vi "RegisterPatchGenerator.vi"(8 "error in":errorcluster, 9 "reg patch file":path=path "C:/Users/liyao/Desktop/New Text Document.Reg", 11 "exe path":path=path "C:/Users/liyao/Desktop/LabVIEW-Version-Selector/Build/LabVIEW Version Selector.exe") -> (0 "error out":errorcluster, 3 "delimited string":string="Windows Registry Editor Version 5.00\n\n[HKEY_CLASSES_ROOT\\Applications\\LabVIEW Version Selector.exe]\n\n[HKEY_CLASSES_ROOT\\Applications\\LabVIEW Version Selector.exe\\shell]\n\n[HKEY_CLASSES_ROOT\\Applications\\LabVIEW Version Selector.exe\\shell\\open]\n\n[HKEY_CLASSES_ROOT\\Applications\\LabVIEW Version Selector.exe\\shell\\open\\command]\n@=\"\\\"\"\"\" \"%1\"\"\\\" \\\"%1\\\"\"\n\n[HKEY_CURRENT_USER\\Software\\Classes\\Applications\\LabVIEW Version Selector.exe]\n\n[HKEY_CURRENT_USER\\Software\\Classes\\Applications\\LabVIEW Version Selector.exe\\shell]\n\n[HKEY_CURRENT_USER\\Software\\Classes\\Applications\\LabVIEW Version Selector.exe\\shell\\open]\n\n[HKEY_CURRENT_USER\\Software\\Classes\\Applications\\LabVIEW Version Selector.exe\\shell\\open\\command]\n@=\"\\\"\"\"\" \"%1\"\"\\\" \\\"%1\\\"\"\n\n[HKEY_CURRENT_USER\\Software\\Microsoft\\Windows\\CurrentVersion\\Explorer\\FileExts\\.lvproj\\OpenWithList]\n\"a\"=\"LabVIEW.exe\"\n\"b\"=\"LabVIEW Version Selector.exe\"\n\"MRUList\"=\"ba\"\n\n[HKEY_CURRENT_USER\\Software\\Microsoft\\Windows\\CurrentVersion\\Explorer\\FileExts\\.lvproj\\UserChoice]\n\"ProgId\"=\"Applications\\\\LabVIEW Version Selector.exe\"\n\n[HKEY_CLASSES_ROOT\\LabVIEWProject\r\n\\shell\\open\\command]\n@=\"\\\"\"\"\" \"%1\"\"\\\" \\\"%1\\\"\"\n\n[HKEY_LOCAL_MACHINE\\SOFTWARE\\Classes\\LabVIEWProject\r\n\\shell\\open\\command]\n@=hex(2):<HEXEXEPATH>\n\n[HKEY_CURRENT_USER\\Software\\Microsoft\\Windows\\CurrentVersion\\Explorer\\FileExts\\.lvlib\\OpenWithList]\n\"a\"=\"LabVIEW.exe\"\n\"b\"=\"LabVIEW Version Selector.exe\"\n\"MRUList\"=\"ba\"\n\n[HKEY_CURRENT_USER\\Software\\Microsoft\\Windows\\CurrentVersion\\Explorer\\FileExts\\.lvlib\\UserChoice]\n\"ProgId\"=\"Applications\\\\LabVIEW Version Selector.exe\"\n\n[HKEY_CLASSES_ROOT\\LabVIEWLabVIEW Library\r\n\\shell\\open\\command]\n@=\"\\\"\"\"\" \"%1\"\"\\\" \\\"%1\\\"\"\n\n[HKEY_LOCAL_MACHINE\\SOFTWARE\\Classes\\LabVIEWLabVIEW Library\r\n\\shell\\open\\command]\n@=hex(2):<HEXEXEPATH>\n\n[HKEY_CURRENT_USER\\Software\\Microsoft\\Windows\\CurrentVersion\\Explorer\\FileExts\\.lvlibp\\OpenWithList]\n\"a\"=\"LabVIEW.exe\"\n\"b\"=\"LabVIEW Version Selector.exe\"\n\"MRUList\"=\"ba\"\n\n[HKEY_CURRENT_USER\\Software\\Microsoft\\Windows\\CurrentVersion\\Explorer\\FileExts\\.lvlibp\\UserChoice]\n\"ProgId\"=\"Applications\\\\LabVIEW Version Selector.exe\"\n\n[HKEY_CLASSES_ROOT\\LabVIEWLabVIEW Packed Library\r\n\\shell\\open\\command]\n@=\"\\\"\"\"\" \"%1\"\"\\\" \\\"%1\\\"\"\n\n[HKEY_LOCAL_MACHINE\\SOFTWARE\\Classes\\LabVIEWLabVIEW Packed Library\r\n\\shell\\open\\command]\n@=hex(2):<HEXEXEPATH>\n\n[HKEY_CURRENT_USER\\Software\\Microsoft\\Windows\\CurrentVersion\\Explorer\\FileExts\\.vi\\OpenWithList]\n\"a\"=\"LabVIEW.exe\"\n\"b\"=\"LabVIEW Version Selector.exe\"\n\"MRUList\"=\"ba\"\n\n[HKEY_CURRENT_USER\\Software\\Microsoft\\Windows\\CurrentVersion\\Explorer\\FileExts\\.vi\\UserChoice]\n\"ProgId\"=\"Applications\\\\LabVIEW Version Selector.exe\"\n\n[HKEY_CLASSES_ROOT\\LabVIEWInstrument\r\n\\shell\\open\\command]\n@=\"\\\"\"\"\" \"%1\"\"\\\" \\\"%1\\\"\"\n\n[HKEY_LOCAL_MACHINE\\SOFTWARE\\Classes\\LabVIEWInstrument\r\n\\shell\\open\\command]\n@=hex(2):<HEXEXEPATH>\n\n[HKEY_CURRENT_USER\\Software\\Microsoft\\Windows\\CurrentVersion\\Explorer\\FileExts\\.llb\\OpenWithList]\n\"a\"=\"LabVIEW.exe\"\n\"b\"=\"LabVIEW Version Selector.exe\"\n\"MRUList\"=\"ba\"\n\n[HKEY_CURRENT_USER\\Software\\Microsoft\\Windows\\CurrentVersion\\Explorer\\FileExts\\.llb\\UserChoice]\n\"ProgId\"=\"Applications\\\\LabVIEW Version Selector.exe\"\n\n[HKEY_CLASSES_ROOT\\LabVIEWLibrary\r\n\\shell\\open\\command]\n@=\"\\\"\"\"\" \"%1\"\"\\\" \\\"%1\\\"\"\n\n[HKEY_LOCAL_MACHINE\\SOFTWARE\\Classes\\LabVIEWLibrary\r\n\\shell\\open\\command]\n@=hex(2):<HEXEXEPATH>\n\n[HKEY_CURRENT_USER\\Software\\Microsoft\\Windows\\CurrentVersion\\Explorer\\FileExts\\.ctl\\OpenWithList]\n\"a\"=\"LabVIEW.exe\"\n\"b\"=\"LabVIEW Version Selector.exe\"\n\"MRUList\"=\"ba\"\n\n[HKEY_CURRENT_USER\\Software\\Microsoft\\Windows\\CurrentVersion\\Explorer\\FileExts\\.ctl\\UserChoice]\n\"ProgId\"=\"Applications\\\\LabVIEW Version Selector.exe\"\n\n[HKEY_CLASSES_ROOT\\LabVIEWControl\r\n\\shell\\open\\command]\n@=\"\\\"\"\"\" \"%1\"\"\\\" \\\"%1\\\"\"\n\n[HKEY_LOCAL_MACHINE\\SOFTWARE\\Classes\\LabVIEWControl\r\n\\shell\\open\\command]\n@=hex(2):<HEXEXEPATH>\n\n[HKEY_CURRENT_USER\\Software\\Microsoft\\Windows\\CurrentVersion\\Explorer\\FileExts\\.lvclass\\OpenWithList]\n\"a\"=\"LabVIEW.exe\"\n\"b\"=\"LabVIEW Version Selector.exe\"\n\"MRUList\"=\"ba\"\n\n[HKEY_CURRENT_USER\\Software\\Microsoft\\Windows\\CurrentVersion\\Explorer\\FileExts\\.lvclass\\UserChoice]\n\"ProgId\"=\"Applications\\\\LabVIEW Version Selector.exe\"\n\n[HKEY_CLASSES_ROOT\\LabVIEWLabVIEW Class\r\n\\shell\\open\\command]\n@=\"\\\"\"\"\" \"%1\"\"\\\" \\\"%1\\\"\"\n\n[HKEY_LOCAL_MACHINE\\SOFTWARE\\Classes\\LabVIEWLabVIEW Class\r\n\\shell\\open\\command]\n@=hex(2):<HEXEXEPATH>\n\n[HKEY_CURRENT_USER\\Software\\Microsoft\\Windows\\CurrentVersion\\Explorer\\FileExts\\.vit\\OpenWithList]\n\"a\"=\"LabVIEW.exe\"\n\"b\"=\"LabVIEW Version Selector.exe\"\n\"MRUList\"=\"ba\"\n\n[HKEY_CURRENT_USER\\Software\\Microsoft\\Windows\\CurrentVersion\\Explorer\\FileExts\\.vit\\UserChoice]\n\"ProgId\"=\"Applications\\\\LabVIEW Version Selector.exe\"\n\n[HKEY_CLASSES_ROOT\\LabVIEWInstrumentTemplate\r\n\\shell\\open\\command]\n@=\"\\\"\"\"\" \"%1\"\"\\\" \\\"%1\\\"\"\n\n[HKEY_LOCAL_MACHINE\\SOFTWARE\\Classes\\LabVIEWInstrumentTemplate\r\n\\shell\\open\\command]\n@=hex(2):<HEXEXEPATH>\n\n[HKEY_CURRENT_USER\\Software\\Microsoft\\Windows\\CurrentVersion\\Explorer\\FileExts\\.xctl\\OpenWithList]\n\"a\"=\"LabVIEW.exe\"\n\"b\"=\"LabVIEW Version Selector.exe\"\n\"MRUList\"=\"ba\"\n\n[HKEY_CURRENT_USER\\Software\\Microsoft\\Windows\\CurrentVersion\\Explorer\\FileExts\\.xctl\\UserChoice]\n\"ProgId\"=\"Applications\\\\LabVIEW Version Selector.exe\"\n\n[HKEY_CLASSES_ROOT\\LabVIEWXControl\r\n\\shell\\open\\command]\n@=\"\\\"\"\"\" \"%1\"\"\\\" \\\"%1\\\"\"\n\n[HKEY_LOCAL_MACHINE\\SOFTWARE\\Classes\\LabVIEWXControl\r\n\\shell\\open\\command]\n@=hex(2):<HEXEXEPATH>\n\n[HKEY_CURRENT_USER\\Software\\Microsoft\\Windows\\CurrentVersion\\Explorer\\FileExts\\.lvtest\\OpenWithList]\n\"a\"=\"LabVIEW.exe\"\n\"b\"=\"LabVIEW Version Selector.exe\"\n\"MRUList\"=\"ba\"\n\n[HKEY_CURRENT_USER\\Software\\Microsoft\\Windows\\CurrentVersion\\Explorer\\FileExts\\.lvtest\\UserChoice]\n\"ProgId\"=\"Applications\\\\LabVIEW Version Selector.exe\"\n\n[HKEY_CLASSES_ROOT\\\\shell\\open\\command]\n@=\"\\\"\"\"\" \"%1\"\"\\\" \\\"%1\\\"\"\n\n[HKEY_LOCAL_MACHINE\\SOFTWARE\\Classes\\\\shell\\open\\command]\n@=hex(2):<HEXEXEPATH>\n\n[HKEY_CURRENT_USER\\Software\\Microsoft\\Windows\\CurrentVersion\\Explorer\\FileExts\\.lvvect\\OpenWithList]\n\"a\"=\"LabVIEW.exe\"\n\"b\"=\"LabVIEW Version Selector.exe\"\n\"MRUList\"=\"ba\"\n\n[HKEY_CURRENT_USER\\Software\\Microsoft\\Windows\\CurrentVersion\\Explorer\\FileExts\\.lvvect\\UserChoice]\n\"ProgId\"=\"Applications\\\\LabVIEW Version Selector.exe\"\n\n[HKEY_CLASSES_ROOT\\\\shell\\open\\command]\n@=\"\\\"\"\"\" \"%1\"\"\\\" \\\"%1\\\"\"\n\n[HKEY_LOCAL_MACHINE\\SOFTWARE\\Classes\\\\shell\\open\\command]\n@=hex(2):<HEXEXEPATH>\n\n[HKEY_CURRENT_USER\\Software\\Microsoft\\Windows\\CurrentVersion\\Explorer\\FileExts\\.lvsc\\OpenWithList]\n\"a\"=\"LabVIEW.exe\"\n\"b\"=\"LabVIEW Version Selector.exe\"\n\"MRUList\"=\"ba\"\n\n[HKEY_CURRENT_USER\\Software\\Microsoft\\Windows\\CurrentVersion\\Explorer\\FileExts\\.lvsc\\UserChoice]\n\"ProgId\"=\"Applications\\\\LabVIEW Version Selector.exe\"\n\n[HKEY_CLASSES_ROOT\\LabVIEW Statechart\r\n\\shell\\open\\command]\n@=\"\\\"\"\"\" \"%1\"\"\\\" \\\"%1\\\"\"\n\n[HKEY_LOCAL_MACHINE\\SOFTWARE\\Classes\\LabVIEW Statechart\r\n\\shell\\open\\command]\n@=hex(2):<HEXEXEPATH>\n\n[HKEY_CURRENT_USER\\Software\\Microsoft\\Windows\\CurrentVersion\\Explorer\\FileExts\\.LVCLASS\\OpenWithList]\n\"a\"=\"LabVIEW.exe\"\n\"b\"=\"LabVIEW Version Selector.exe\"\n\"MRUList\"=\"ba\"\n\n[HKEY_CURRENT_USER\\Software\\Microsoft\\Windows\\CurrentVersion\\Explorer\\FileExts\\.LVCLASS\\UserChoice]\n\"ProgId\"=\"Applications\\\\LabVIEW Version Selector.exe\"\n\n[HKEY_CLASSES_ROOT\\LabVIEWLabVIEW Class\r\n\\shell\\open\\command]\n@=\"\\\"\"\"\" \"%1\"\"\\\" \\\"%1\\\"\"\n\n[HKEY_LOCAL_MACHINE\\SOFTWARE\\Classes\\LabVIEWLabVIEW Class\r\n\\shell\\open\\command]\n@=hex(2):<HEXEXEPATH>\n\n[HKEY_CURRENT_USER\\Software\\Microsoft\\Windows\\CurrentVersion\\Explorer\\FileExts\\.lvr\\OpenWithList]\n\"a\"=\"LabVIEW.exe\"\n\"b\"=\"LabVIEW Version Selector.exe\"\n\"MRUList\"=\"ba\"\n\n[HKEY_CURRENT_USER\\Software\\Microsoft\\Windows\\CurrentVersion\\Explorer\\FileExts\\.lvr\\UserChoice]\n\"ProgId\"=\"Applications\\\\LabVIEW Version Selector.exe\"\n\n[HKEY_CLASSES_ROOT\\\\shell\\open\\command]\n@=\"\\\"\"\"\" \"%1\"\"\\\" \\\"%1\\\"\"\n\n[HKEY_LOCAL_MACHINE\\SOFTWARE\\Classes\\\\shell\\open\\command]\n@=hex(2):<HEXEXEPATH>\n\n[HKEY_CURRENT_USER\\Software\\Microsoft\\Windows\\CurrentVersion\\Explorer\\FileExts\\.lvrbt\\OpenWithList]\n\"a\"=\"LabVIEW.exe\"\n\"b\"=\"LabVIEW Version Selector.exe\"\n\"MRUList\"=\"ba\"\n\n[HKEY_CURRENT_USER\\Software\\Microsoft\\Windows\\CurrentVersion\\Explorer\\FileExts\\.lvrbt\\UserChoice]\n\"ProgId\"=\"Applications\\\\LabVIEW Version Selector.exe\"\n\n[HKEY_CLASSES_ROOT\\LabVIEWNXTRobotProject\r\n\\shell\\open\\command]\n@=\"\\\"\"\"\" \"%1\"\"\\\" \\\"%1\\\"\"\n\n[HKEY_LOCAL_MACHINE\\SOFTWARE\\Classes\\LabVIEWNXTRobotProject\r\n\\shell\\open\\command]\n@=hex(2):<HEXEXEPATH>")   [LabVIEW 2014]
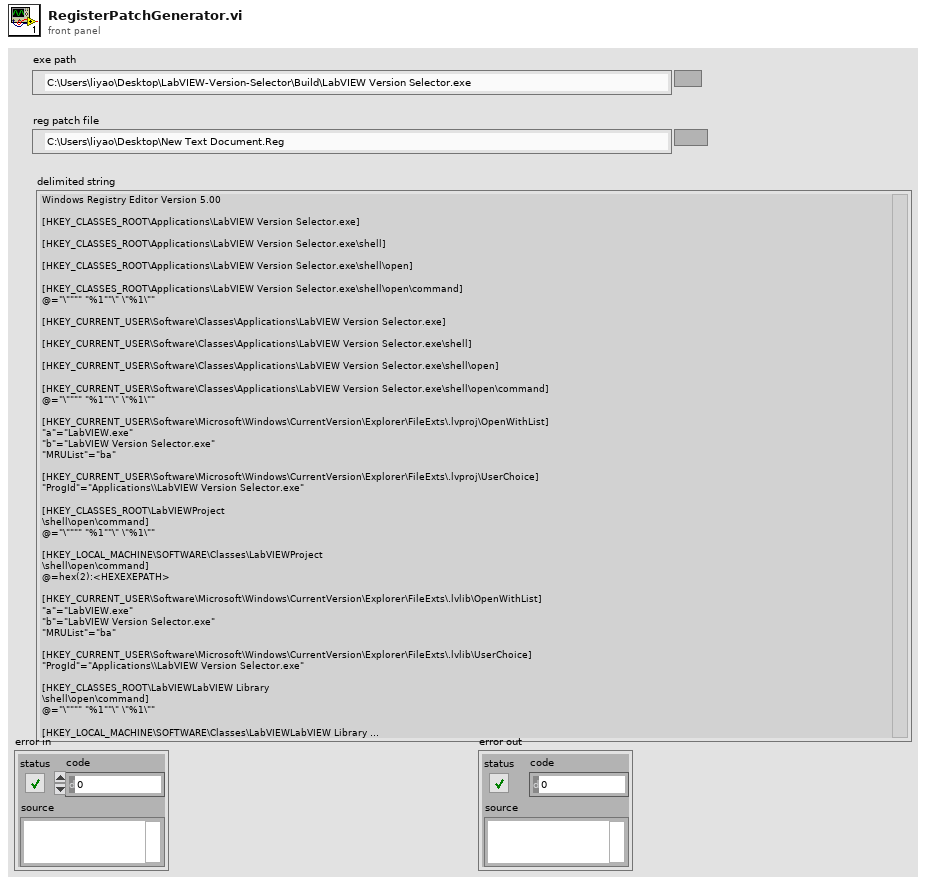
[diagram p1: front panel]
types:
  T1 = enum16{"open", "replace", "create", "open or create", "replace or create", "replace or create with confirmation"}
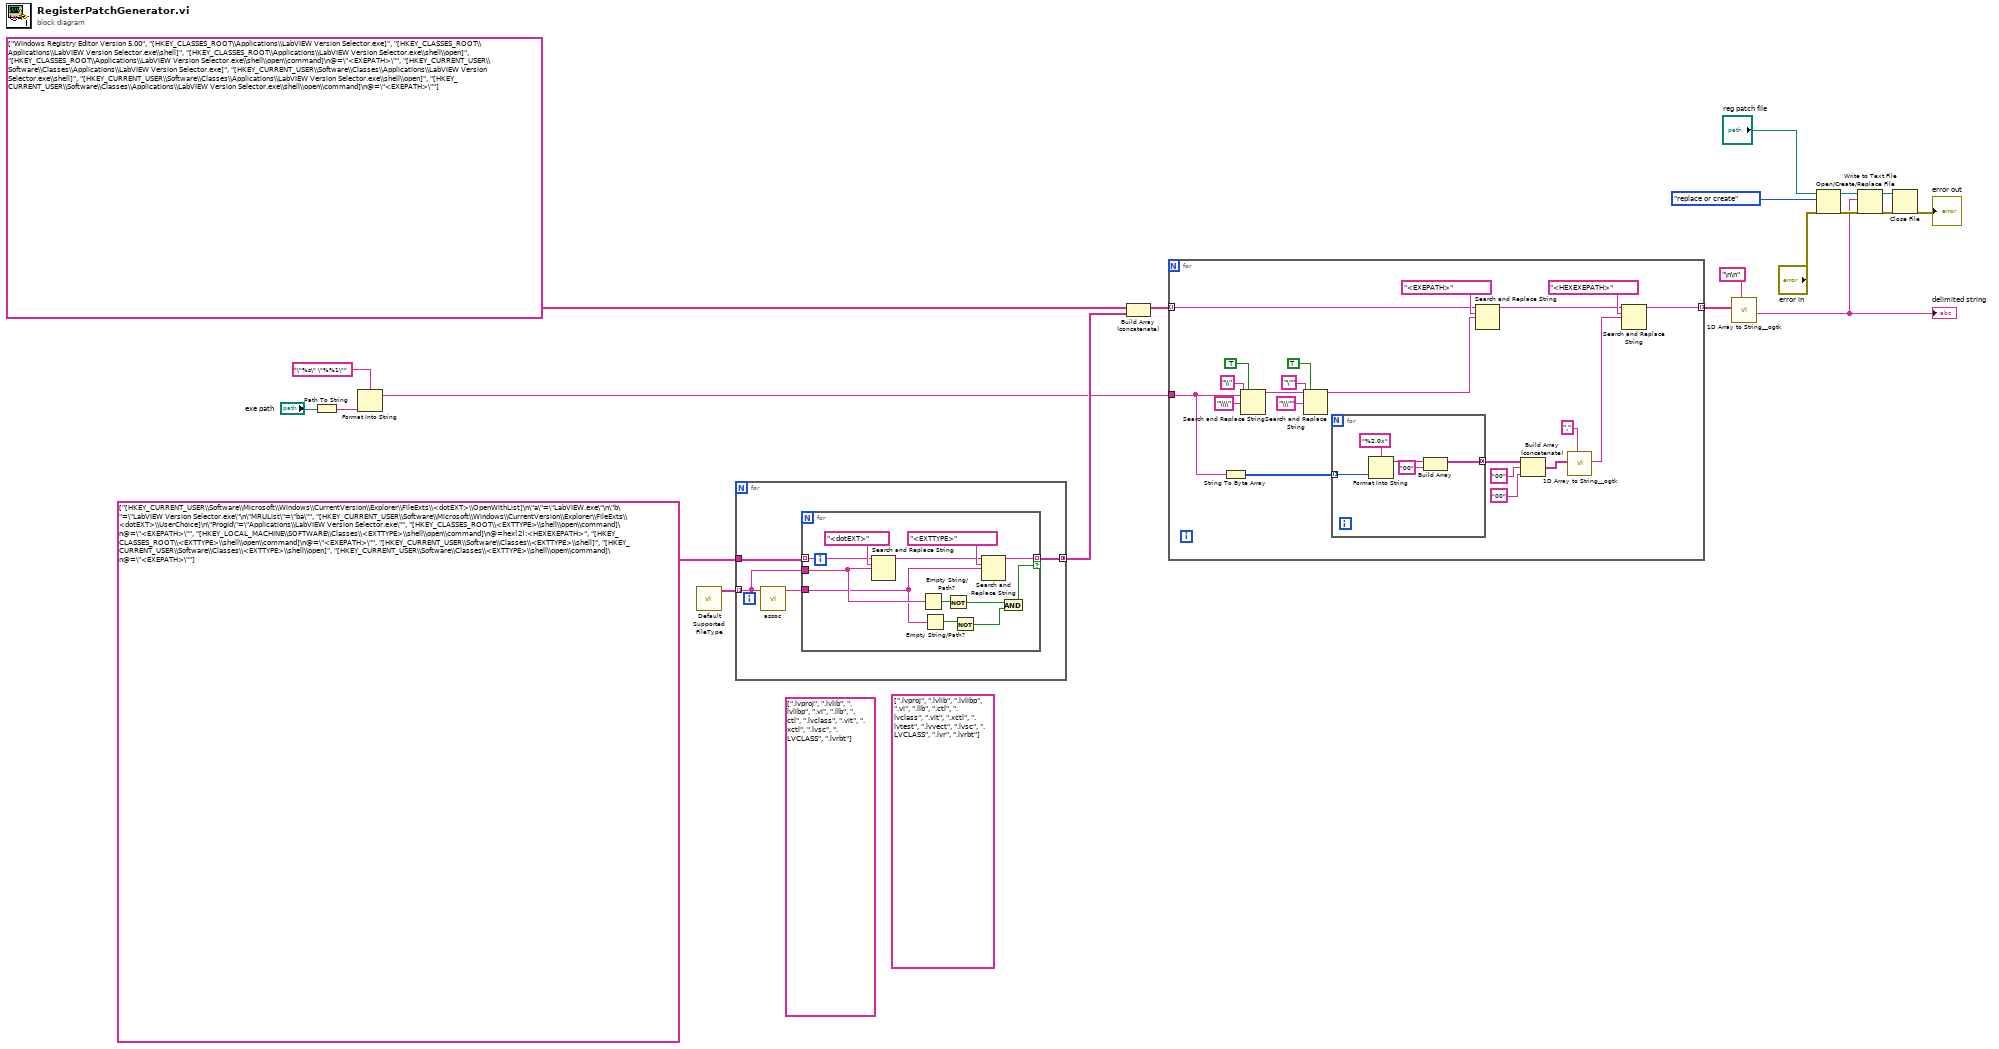
[diagram p0: block diagram]
diagram:
  (unwired) string[] [".lvproj", ".lvlib", ".lvlibp", ".vi", ".llb", ".ctl", ".lvclass", ".vit", ".xctl", ".lvtest", ".lvvect", ".lvsc", ".LVCLASS", ".lvr", ".lvrbt"] ("Array")
  (unwired) string[] [".lvproj", ".lvlib", ".lvlibp", ".vi", ".llb", ".ctl", ".lvclass", ".vit", ".xctl", ".lvsc", ".LVCLASS", ".lvrbt"] ("Array")
  n1 = Path To String(path="exe path") -> (string=w12:string)
  n2 = Format Into String(format string="\"%s\" \"%%1\"", w12) -> (resulting string=w11:string)  [unwired: 2 in, 1 out]
  n3 = call "Default Supported FileType.vi"() -> ("Array"=w1:string[])  [unwired: 11 in]
  n4 = for {
    tunnel: string[] ["[HKEY_CURRENT_USER\\Software\\Microsoft\\Windows\\CurrentVersion\\Explorer\\FileExts\\<dotEXT>\\OpenWithList]\n\"a\"=\"LabVIEW.exe\"\n\"b\"=\"LabVIEW Version Selector.exe\"\n\"MRUList\"=\"ba\"", "[HKEY_CURRENT_USER\\Software\\Microsoft\\Windows\\CurrentVersion\\Explorer\\FileExts\\<dotEXT>\\UserChoice]\n\"ProgId\"=\"Applications\\LabVIEW Version Selector.exe\"", "[HKEY_CLASSES_ROOT\\<EXTTYPE>\\shell\\open\\command]\n@=\"<EXEPATH>\"", "[HKEY_LOCAL_MACHINE\\SOFTWARE\\Classes\\<EXTTYPE>\\shell\\open\\command]\n@=hex(2):<HEXEXEPATH>", "[HKEY_CLASSES_ROOT\\<EXTTYPE>\\shell\\open\\command]\n@=\"<EXEPATH>\"", "[HKEY_CURRENT_USER\\Software\\Classes\\<EXTTYPE>\\shell]", "[HKEY_CURRENT_USER\\Software\\Classes\\<EXTTYPE>\\shell\\open]", "[HKEY_CURRENT_USER\\Software\\Classes\\<EXTTYPE>\\shell\\open\\command]\n@=\"<EXEPATH>\""] -> [w24]
    tunnel: w1 -> [w22] mode=indexing
    tunnel: [w21] -> w14 mode=concatenating
    n5 = call "assoc.vi"("input 1"=w22) -> ("standard output"=w23:string)  [unwired: 10 in]
    n6 = for {
      tunnel: w24 -> [w32] mode=indexing
      tunnel: [w33] -> w21 mode=indexing if=w27
      tunnel: w22 -> [w26]
      tunnel: w23 -> [w25]
      n7 = Search and Replace String(input string=w32, search string="<dotEXT>", replace string=w26) -> (result string=w34:string)  [unwired: 5 in, 3 out]
      n8 = Empty String/Path?(string/path=w26) -> (empty?=w31:bool)
      n9 = Empty String/Path?(string/path=w25) -> (empty?=w30:bool)
      n10 = Not(x=w31) -> (.not. x?=w28:bool)
      n11 = Not(x=w30) -> (.not. x?=w29:bool)
      n12 = Search and Replace String(input string=w34, search string="<EXTTYPE>", replace string=w25) -> (result string=w33:string)  [unwired: 5 in, 3 out]
      n13 = And(x=w28, y=w29) -> (x .and. y?=w27:bool)
    }
  }
  n14 = Build Array (concatenate)(string[] ["Windows Registry Editor Version 5.00", "[HKEY_CLASSES_ROOT\\Applications\\LabVIEW Version Selector.exe]", "[HKEY_CLASSES_ROOT\\Applications\\LabVIEW Version Selector.exe\\shell]", "[HKEY_CLASSES_ROOT\\Applications\\LabVIEW Version Selector.exe\\shell\\open]", "[HKEY_CLASSES_ROOT\\Applications\\LabVIEW Version Selector.exe\\shell\\open\\command]\n@=\"<EXEPATH>\"", "[HKEY_CURRENT_USER\\Software\\Classes\\Applications\\LabVIEW Version Selector.exe]", "[HKEY_CURRENT_USER\\Software\\Classes\\Applications\\LabVIEW Version Selector.exe\\shell]", "[HKEY_CURRENT_USER\\Software\\Classes\\Applications\\LabVIEW Version Selector.exe\\shell\\open]", "[HKEY_CURRENT_USER\\Software\\Classes\\Applications\\LabVIEW Version Selector.exe\\shell\\open\\command]\n@=\"<EXEPATH>\""], w14) -> (w15:string[])
  n15 = for {
    tunnel: w15 -> [w56] mode=indexing
    tunnel: w11 -> [w48]
    tunnel: [w50] -> w18 mode=indexing
    n16 = String To Byte Array(string=w48) -> (unsigned byte array=w47:u8[])
    n17 = Search and Replace String(replace all?=TRUE ("replace all? (F)"), input string=w48, search string="\\", replace string="\\\\" ("replace string (\"\")")) -> (result string=w38:string)  [unwired: 4 in, 3 out]
    n18 = Search and Replace String(replace all?=TRUE ("replace all? (F)"), input string=w38, search string="\"", replace string="\\\"" ("replace string (\"\")")) -> (result string=w37:string)  [unwired: 4 in, 3 out]
    n19 = for {
      tunnel: [w59] -> w49 mode=concatenating
      tunnel: w47 -> [w62] mode=indexing
      n20 = Format Into String(format string="%2.0x", w62) -> (resulting string=w60:string)  [unwired: 2 in, 1 out]
      n21 = Build Array(w60, "00" ("element")) -> (w59:string[])
    }
    n22 = Search and Replace String(input string=w56, search string="<EXEPATH>", replace string=w37) -> (result string=w51:string)  [unwired: 5 in, 3 out]
    n23 = Build Array (concatenate)(w49, "00" ("element"), "00" ("element")) -> (w44:string[])
    n24 = call <userlib>:"1D Array to String__ogtk.vi"("delimiter (Tab)"=",", "Array of Strings"=w44) -> ("delimited string"=w46:string)  [unwired: 9 in]
    n25 = Search and Replace String(input string=w51, search string="<HEXEXEPATH>", replace string=w46) -> (result string=w50:string)  [unwired: 5 in, 3 out]
  }
  n26 = call <userlib>:"1D Array to String__ogtk.vi"("delimiter (Tab)"="\n\n", "Array of Strings"=w18) -> ("delimited string"=w4:string)  [unwired: 9 in]
  "delimited string" <- w4
  n27 = Open/Create/Replace File(file path (use dialog)="reg patch file", error in="error in", operation (0:open)=T1."replace or create") -> (refnum out=w8:refnum<file>, error out=w5:errorcluster)  [unwired: 3 in, 1 out]
  n28 = Write to Text File(file (use dialog)=w8, text=w4, error in=w5) -> (refnum out=w7:refnum<file>, error out=w6:errorcluster)  [unwired: 1 in, 1 out]
  n29 = Close File(refnum=w7, error in=w6) -> (error out=→"error out":errorcluster)  [unwired: 1 out]
